vi "Test Update 1.vi"(11 "Test Case In":refnum<class "Camera Tests.lvclass">) -> (0 "error out":errorcluster, 3 "Test Case Out":refnum<class "Camera Tests.lvclass">)   [LabVIEW 2021, in "Camera Tests.lvclass"]
uses:
  Camera Tests.lvclass
  4993e8ee-a06a-463a-9684-69129f64d5ce.vi
  Application Specific/Camera/Camera.lvclass
  Re-use Libraries/Vector 2D/Vector 2D.lvclass
  e086f2d9-95d8-4aa4-9347-c0290e2d8edc.vi
  b405ea4c-2126-4b06-9b15-9c90e9a4e760.vi
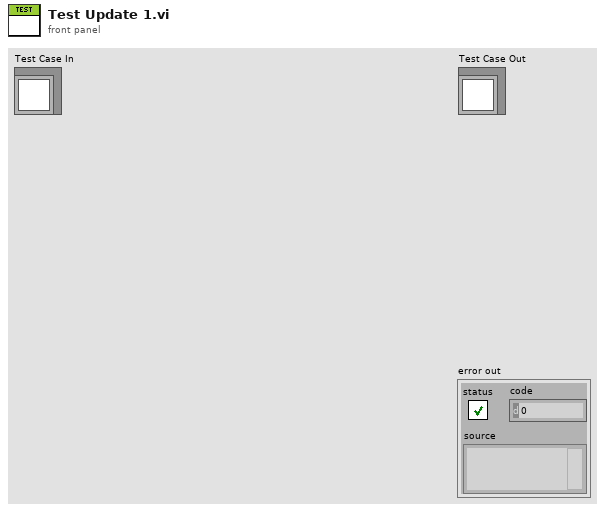
[diagram p1: front panel]
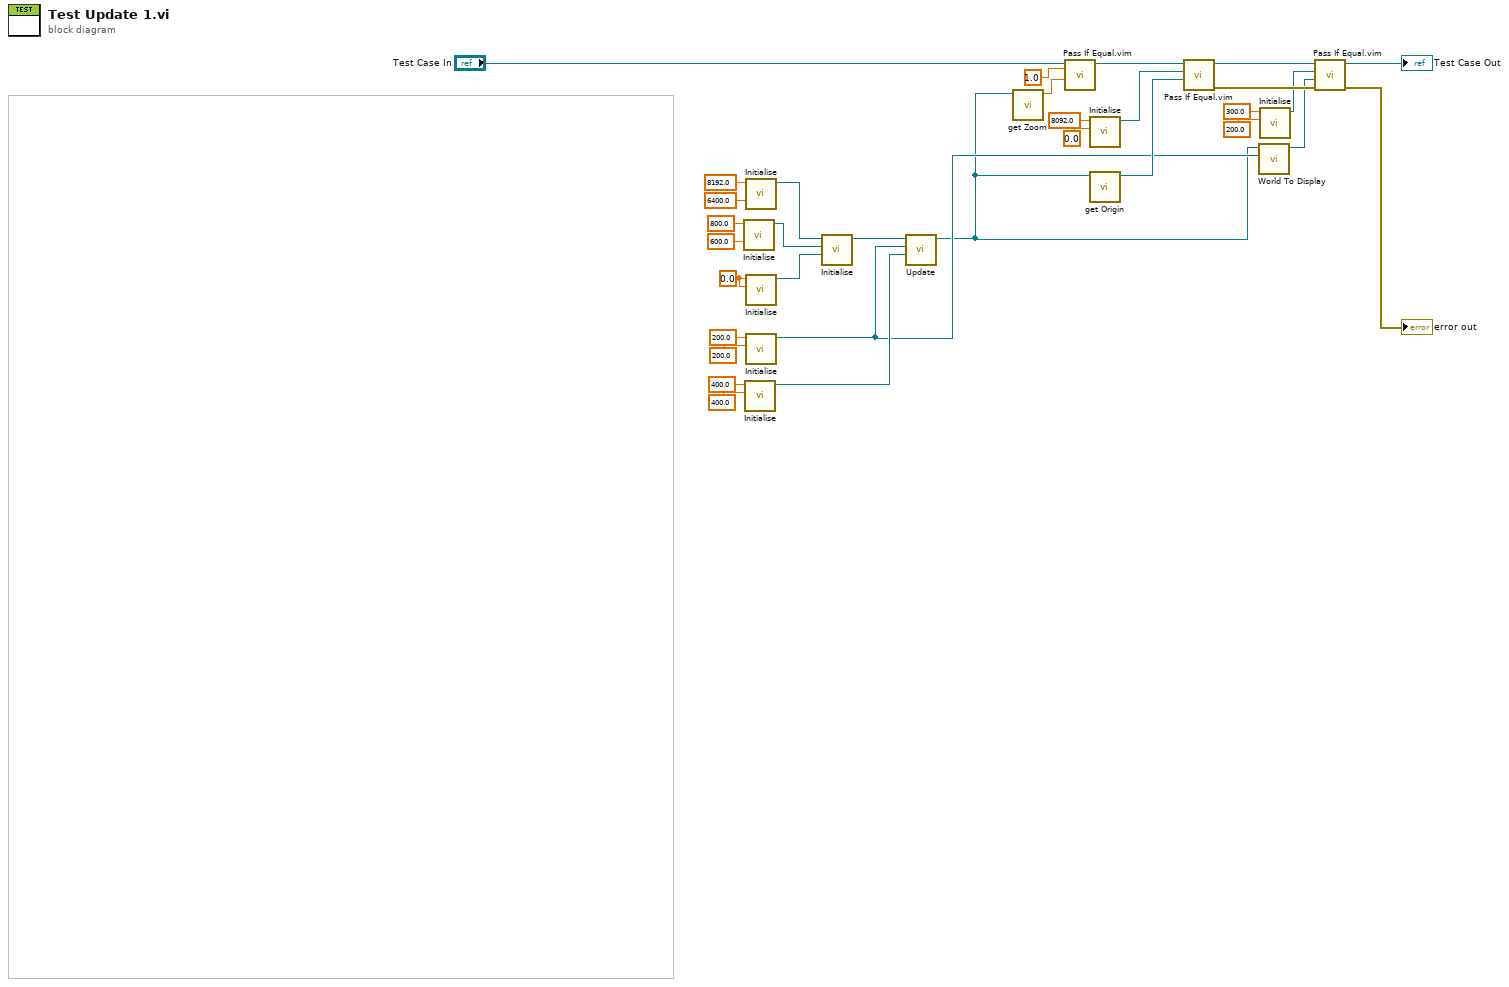
[diagram p0: block diagram]
diagram:
  w29 = sgl 0.0 ("x")
  n1 = call "Initialise.vi"("y"=sgl 600.0, "x"=sgl 800.0) -> ("Vector 2D out"=w7:refnum<class "Vector 2D.lvclass">)  [unwired: 9 in]
  n2 = call "Initialise.vi"("y"=sgl 400.0, "x"=sgl 400.0) -> ("Vector 2D out"=w22:refnum<class "Vector 2D.lvclass">)  [unwired: 9 in]
  n3 = call "Initialise.vi"("y"=sgl 6400.0, "x"=sgl 8192.0) -> ("Vector 2D out"=w30:refnum<class "Vector 2D.lvclass">)  [unwired: 9 in]
  n4 = call "Initialise.vi"("y"=w29, "x"=w29) -> ("Vector 2D out"=w28:refnum<class "Vector 2D.lvclass">)  [unwired: 9 in]
  n5 = call "Initialise.vi"("y"=sgl 200.0, "x"=sgl 200.0) -> ("Vector 2D out"=w13:refnum<class "Vector 2D.lvclass">)  [unwired: 9 in]
  n6 = call "Initialise.vi"("Origin"=w28, "View Size"=w7, "World Size"=w30) -> ("Camera out"=w23:refnum<class "Camera.lvclass">)  [unwired: 8 in]
  n7 = call "Update.vi"("Player 2 Position"=w22, "Player 1 Position"=w13, "Camera in"=w23) -> ("Camera out"=w2:refnum<class "Camera.lvclass">)  [unwired: 8 in]
  n8 = call "get Zoom.vi"("Camera in"=w2) -> ("Zoom Level"=w6:sgl)  [unwired: 10 in]
  n9 = call "Pass If Equal.vim"("Actual"=w6, "Expected"=sgl 1.0 ("Zoom Level"), "LUnit Test Case In"="Test Case In") -> ("LUnit Test Case Out"=w3:refnum<class "Camera Tests.lvclass">)  [unwired: 7 in, 1 out]
  n10 = call "Initialise.vi"("y"=sgl 0.0, "x"=sgl 8092.0) -> ("Vector 2D out"=w18:refnum<class "Vector 2D.lvclass">)  [unwired: 9 in]
  n11 = call "get Origin.vi"("Camera in"=w2) -> ("Origin"=w21:refnum<class "Vector 2D.lvclass">)  [unwired: 10 in]
  n12 = call "Pass If Equal.vim"("Actual"=w21, "Expected"=w18, "LUnit Test Case In"=w3) -> ("error out"=w15:errorcluster, "LUnit Test Case Out"=w17:refnum<class "Camera Tests.lvclass">)  [unwired: 7 in]
  n13 = call "World To Display.vi"("World Position"=w13, "Camera in"=w2) -> ("Display Position"=w9:refnum<class "Vector 2D.lvclass">)  [unwired: 9 in]
  n14 = call "Initialise.vi"("y"=sgl 200.0, "x"=sgl 300.0) -> ("Vector 2D out"=w10:refnum<class "Vector 2D.lvclass">)  [unwired: 9 in]
  n15 = call "Pass If Equal.vim"("error in (no error)"=w15, "Actual"=w9, "Expected"=w10, "LUnit Test Case In"=w17) -> ("error out"=→"error out":errorcluster, "LUnit Test Case Out"=→"Test Case Out":refnum<class "Camera Tests.lvclass">)  [unwired: 6 in]
